vi "Log Output.vi"(6 "VI Name":string, 7 "error in (no error)":errorcluster caption="エラー入力 (エラーなし)" {"code" format="%.0x"}) -> (0 "error out":errorcluster caption="エラー出力" {"code" format="%.0x"})   [LabVIEW 2014]
panel:
  out "Appending Strings(debug)":string
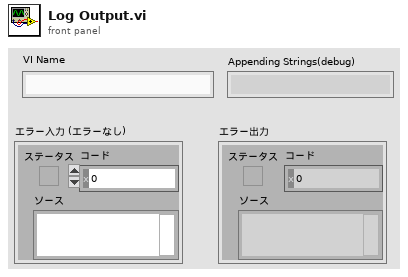
[diagram p1: front panel]
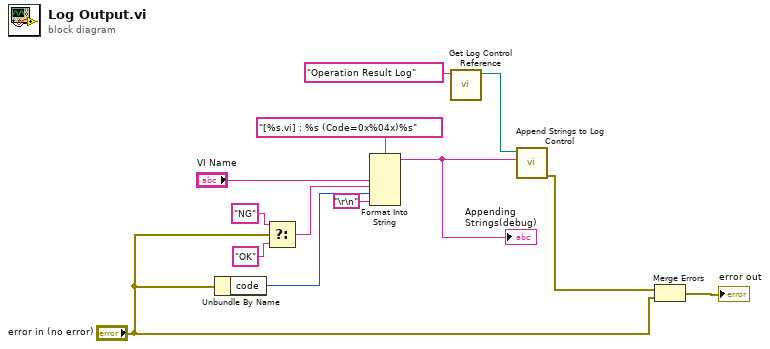
[diagram p0: block diagram]
diagram:
  n1 = Unbundle By Name("error in (no error)") -> ("code"=w8:i32)
  n2 = Select(t="NG" ("Œ`Ž®•¶Žš—ñ"), s="error in (no error)", f="OK" ("Œ`Ž®•¶Žš—ñ")) -> (s? t:f=w9:string)
  n3 = Format Into String(format string="[%s.vi] : %s (Code=0x%04x)%s" ("Œ`Ž®•¶Žš—ñ"), "VI Name", w9, w8, "\r\n") -> (resulting string=w5:string)  [unwired: 2 in, 1 out]
  "Appending Strings(debug)" <- w5
  n4 = call "Get Log Control Reference.vi"("Log Control  Name"="Operation Result Log") -> ("Referece to Log Control"=w4:refnum<vi>)  [unwired: 9 in, 1 out]
  n5 = call "Append Strings to Log Control.vi"("Appending Strings"=w5, "Reference to Log Control"=w4) -> ("エラー出力"=w2:errorcluster)  [unwired: 9 in]
  n6 = Merge Errors(w2, "error in (no error)") -> (→"error out":errorcluster)
